vi "Soma.vi"(10 "y":dbl, 11 "x":dbl) -> (2 "(x+10)*y":dbl, 3 "x+10":dbl)   [LabVIEW 2018]
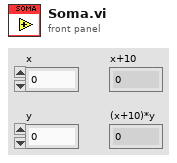
[diagram p1: front panel]
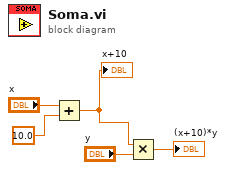
[diagram p0: block diagram]
diagram:
  n1 = Add(x="x", y=10.0) -> (x+y=w5:dbl)
  "x+10" <- w5
  n2 = Multiply(x=w5, y="y") -> (x*y=→"(x+10)*y":dbl)
